vi "dsdata.vi"() -> ()   [LabVIEW 2019]
doc: "This global variable contains data from the FMS system as well as the FRC 4265 Dashboard including safety overrides, calibration commands, and configuration parameters. These data are updated during all robot modes. Robot commands should never be placed in this global variable."
uses:
  <vilib>/Rock Robotics/WPI/DriverStation/WPI_DriverStationRobotMode2.ctl
panel:
  out "Running_Systems_Check":bool
  out "New_Driver_Profile_Setpoints":dbl[](array[numeric])
  out "Apply_Driver_Profile_Setpoints":bool
  out "Starting_Safety_Override":bool
  out "Starting_IMU_Reset":bool
  out "Apply_New_Shooter_Setpoint":bool
  out "Selected_Shooter_Setpoint_Index":i32
  out "New_Shooter_Setpoint (rpm)":dbl
  out "Field_Oriented_Override":bool
  out "Driver_DPad":T1(ring)
  out "Selected_Default_Pipeline":T2(ring)=enum."Power Port"
  out "Force_Human_Control":bool
  out "Selected_Robot":i32
  out "Test_Actuator_Period (s)":dbl
  out "Driver_Joystick_Calibrations":dbl[](array[numeric])
  out "Calibrate_Joysticks":bool
  out "Robot_is_Autonomous":bool
  out "Master_Caution":bool
  out "Starting_Tablet_Override":bool
  out "Tablet_Override":bool
  out "Auto_Target_Override":bool
  out "Test_Actuator_Value":dbl
  out "Test_Actuator_Name":string
  out "Disable_Fusion_Y":bool
  out "Disable_Fusion_X":bool
  out "Camera_Override":bool
  out "Auto_Test_Mode":bool
  out "Clear_Errors":bool
  out "Master_Safety_Override":bool
  out "Auto_Delay (s)":dbl
  out "Zero_Wheels":bool
  out "Calibrate_Wheels":bool
  out "Selected_Driver":i32
  out "Tune_Tab":bool
  out "Selected_Auto_Play":u16
  out "Refresh_Auto_Play_List":bool
  out "Super_Test_Mode":bool
  out "Robot Mode":T3
  # "--FMS--"
  # "--driver joystick--"
  # "--setup and auto--"
  # "--overrides--"
  # "--tune tab--"
  # "--calculations performed on driver station--"
  # "--drivebase tuning--"
  # "--shooter tuning--"
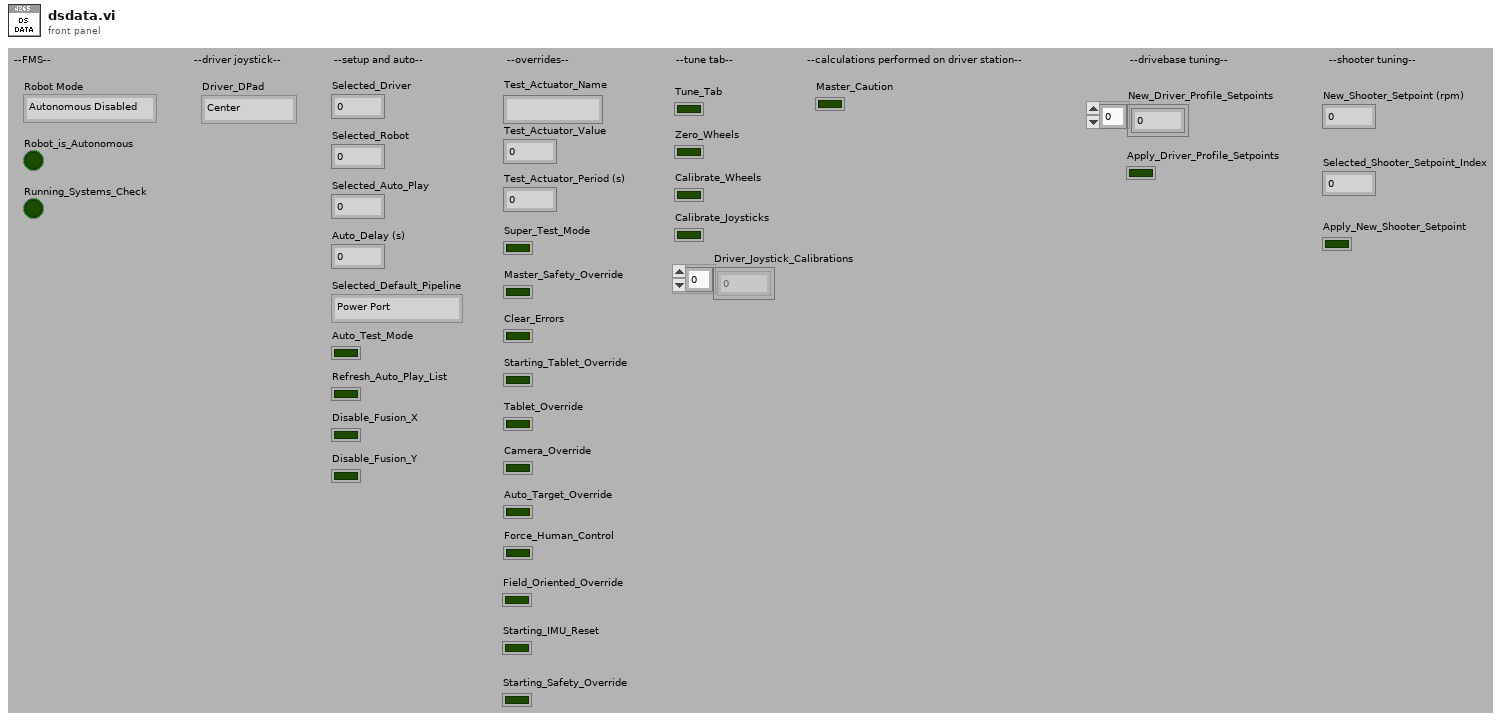
[diagram p1: front panel]
types:
  T1 = enum16{"Center", "North", "NorthWest", "West", "SouthWest", "South", "SouthEast", "East", "NorthEast"}
  T2 = enum16{"Boot Up", "Camera Override", "Power Port", "Ball Tracking"}
  T3 = typedef "WPI_DriverStationRobotMode2.ctl" = enum16{"Autonomous Disabled", "Autonomous Enabled", "Teleop Disabled", "Teleop Enabled", "Disconnected", "Finish", "Test Disabled", "Test Enabled", "Emergency Stopped"}
diagram:
